vi "Get Device Info.vi"(8 "error in (no error)":errorcluster, 11 "RIO Device":T1) -> (0 "error out":errorcluster, 1 "SI Channels":string[](array[string]), 2 "SI Count":i32, 3 "Module Name":string)   [LabVIEW 2025]
uses:
  <vilib>/userDefined/Silver/nirio_resource_slv.ctl
  <vilib>/nisyscfg/Close (System).vi
  Error Strings Global Internal.vi
  <vilib>/nisyscfg/nisyscfg.lvlib
  <resource>/objmgr/niflexrioatomicsae.rc
  <resource>/objmgr/nicriosae.rc
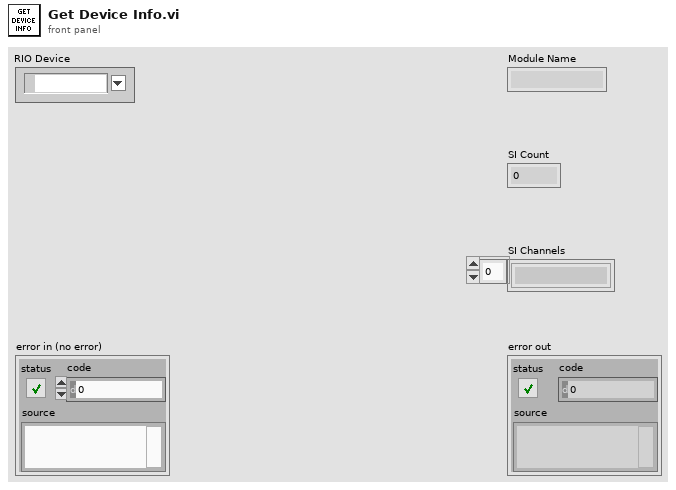
[diagram p1: front panel]
types:
  T1 = typedef "nirio_resource_slv.ctl" = tag
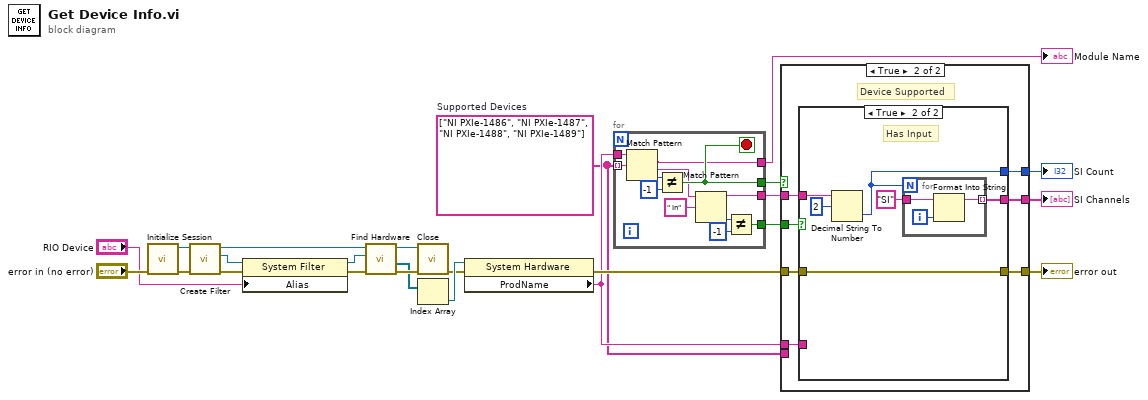
[diagram p0: block diagram]
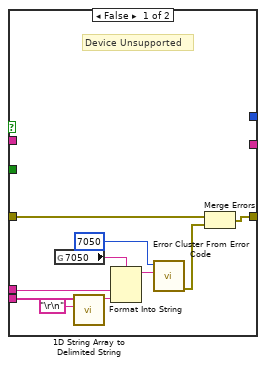
[diagram p2: hidden frame]
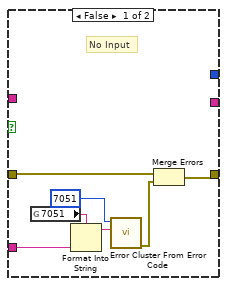
[diagram p3: hidden frame]
diagram:
  w1 = string[] ["NI PXIe-1486", "NI PXIe-1487", "NI PXIe-1488", "NI PXIe-1489"]  # Supported Devices
  n1 = call <vilib>:"Initialize Session.vi"("error in (no error)"="error in (no error)") -> ("error out"=w14:errorcluster, "Session out"=w12:refnum<k21>)  [unwired: 9 in]
  n2 = call <vilib>:"Create Filter.vi"("error in (no error)"=w14, "Session in"=w12) -> ("error out"=w9:errorcluster, "Filter out"=w10:refnum<k20>, "Session out"=w13:refnum<k21>)  [unwired: 7 in]
  n3 = property class="System Filter"(reference=w10, error in=w9, "Alias"="RIO Device") -> (reference out=w11:refnum<k20>, error out=w15:errorcluster)
  n4 = call <vilib>:"Find Hardware.vi"("error in (no error)"=w15, "Filter in"=w11, "Session in"=w13) -> ("error out"=w18:errorcluster, "Resources out"=w8:refnum<k20>[], "Session out"=w7:refnum<k21>)  [unwired: 5 in, 1 out]
  n5 = call-poly <vilib>:"Close.vi"("error in (no error)"=w18, "Session in"=w7) -> ("error out"=w6:errorcluster)  [unwired: 9 in]
  n6 = Index Array(array=w8) -> (element=w17:refnum<k20>)  [unwired: 1 in]
  n7 = property class="System Hardware"(reference=w17, error in=w6) -> (error out=w5:errorcluster, "ProdName"=w2:string)  [unwired: 1 out]
  n8 = for {
    tunnel: w1 -> [w30] mode=indexing
    tunnel: w2 -> [w36]
    tunnel: [w33] -> w4
    tunnel: [w29] -> w22
    tunnel: [w27] -> w19
    tunnel: [w26] -> w21
    stop <- w33 stop-if-true
    n9 = Match Pattern(string=w36, regular expression=w30) -> (match substring=w29:string, after substring=w25:string, offset past match=w35:i32)  [unwired: 1 in, 1 out]
    n10 = Not Equal?(x=w35, y=-1) -> (x != y?=w33:bool)
    n11 = Match Pattern(string=w25, regular expression=" In") -> (before substring=w27:string, offset past match=w31:i32)  [unwired: 1 in, 2 out]
    n12 = Not Equal?(x=w31, y=-1) -> (x != y?=w26:bool)
  }
  "Module Name" <- w22
  n13 = case shown="True" w4 {
    tunnel: [_ w53] -> w23
    tunnel: w21 -> [_ w52]
    tunnel: [_ w51] -> w20
    tunnel: w19 -> [_ w50]
    tunnel: w5 -> [w39 w49]
    tunnel: [w38 w48] -> w3
    tunnel: w2 -> [w45 w47]
    tunnel: w1 -> [w44 _]
    frame False {
      # "Device Unsupported"
      n14 = global read "Error Strings Global Internal.vi" "7050"() -> (w46:string)
      n15 = call <vilib>:"1D String Array to Delimited String.vi"("delimiter"="\r\n", "string array"=w44) -> ("delimited string"=w42:string)  [unwired: 9 in]
      n16 = Format Into String(format string=w46, w45, w42) -> (resulting string=w41:string)  [unwired: 2 in, 1 out]
      n17 = call <vilib>:"Error Cluster From Error Code.vi"("error message (\"\")"=w41, "error code (0)"=7050) -> ("error out"=w37:errorcluster)  [unwired: 7 in]
      n18 = Merge Errors(w39, w37) -> (w38:errorcluster)
    }
    frame True {
      # "Device Supported"
      n19 = case shown="True" w52 {
        tunnel: w50 -> [_ w66]
        tunnel: [_ w64] -> w53
        tunnel: [_ w62] -> w51
        tunnel: w49 -> [w55 w61]
        tunnel: [w54 w61] -> w48
        tunnel: w47 -> [w56 _]
        frame False {
          # "No Input"
          n20 = global read "Error Strings Global Internal.vi" "7051"() -> (w60:string)
          n21 = Format Into String(format string=w60, w56) -> (resulting string=w59:string)  [unwired: 2 in, 1 out]
          n22 = call <vilib>:"Error Cluster From Error Code.vi"("error message (\"\")"=w59, "error code (0)"=7051) -> ("error out"=w57:errorcluster)  [unwired: 7 in]
          n23 = Merge Errors(w55, w57) -> (w54:errorcluster)
        }
        frame True {
          # "Has Input"
          n24 = Decimal String To Number(string=w66, offset=2) -> (number=w64:i32)  [unwired: 1 in, 1 out]
          n25 = for {
            N: w64 -> [_]
            tunnel: "SI" -> [w69]
            tunnel: [w67] -> w62 mode=indexing
            i -> [w68]
            n26 = Format Into String(initial string=w69, w68) -> (resulting string=w67:string)  [unwired: 2 in, 1 out]
          }
        }
      }
    }
  }
  "error out" <- w3
  "SI Count" <- w23
  "SI Channels" <- w20
